vi "OAT Orbit Plot (Angle Waveform).vi"(0 "angle waveform (X and Y)":cluster{"r0":dbl, "dr":dbl, "Y":dbl[]}[](array[cluster]) {"r0" format="%.2p"; "dr" format="%.2p"; "Y" format="%.2f"}, 1 "orbit plot ref":refnum<vi>, 2 "reset? (T)":bool=TRUE, 3 "max axis display value":dbl format="%.2f", 5 "speed profile":T1 {"speed [RPM]" format="%.2f"; "time [s]" format="%.2f"}, 7 "interpolated pulse positions [s]":dbl[](array[numeric]) format="%.2f", 9 "revolutions to display":cluster{"start [rev]":dbl, "duration [rev]":dbl}={"start [rev]"=0.0, "duration [rev]"=1.0} {"duration [rev]" format="%.2f"; "start [rev]" format="%.2f"}, 11 "error in (no error)":errorcluster, 12 "rotating settings":T2={"shaft rotating direction"=0, "probe orientation"={"X (red)"=0, "Y (blue)"=90}} {"shaft rotating direction" items=["CCW", "CW"]}, 14 "trigger pulse direction":u16(ring)=1 items=["positive going", "negative going"]) -> (4 "orbit plot":T3, 15 "error out":errorcluster)   [LabVIEW 2017]
doc: "Draws an orbit plot of waveform signals on an XY graph. You can use sampled or resampled waveform signals from proximity transducers. You can use this polymorphic VI to draw an orbit plot of resampled signals or waveform signals. The data type you wire to the <B>resampled signals (X and Y)</B> determines the polymorphic instance to use."
uses:
  <vilib>/addons/Sound and Vibration/Order Analysis/Backward Compatibility/SubVIs/oa_Orbit Plot Control.ctl
  <vilib>/addons/Sound and Vibration/Order Analysis/Tach Process/SubVIs/speed profile.ctl
  <vilib>/addons/Sound and Vibration/Order Analysis/Resample Order Tracking/SoundVib_Resampling.lvlib
  <vilib>/addons/Sound and Vibration/Order Analysis/Tach Process/SoundVib_TachProcess.lvlib
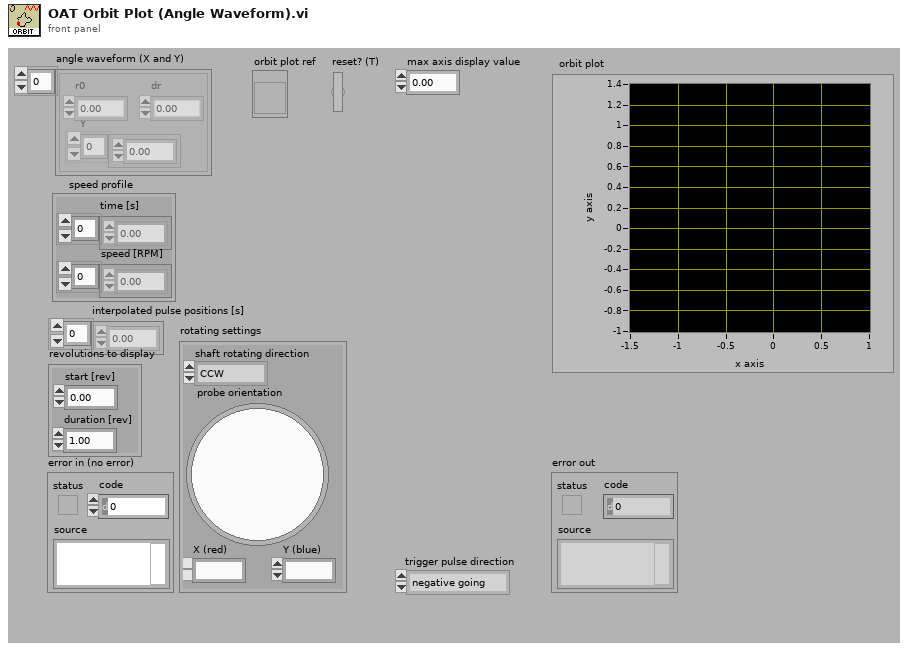
[diagram p1: front panel]
types:
  T1 = typedef "SoundVib_TachProcess.lvlib/speed profile.ctl" = cluster{"time [s]":dbl[], "speed [RPM]":dbl[]}
  T2 = cluster{"shaft rotating direction":u16, "probe orientation":cluster{"X (red)":u32, "Y (blue)":u32}}
  T3 = typedef "oa_Orbit Plot Control.ctl" = cluster{dbl[], dbl[]}[]
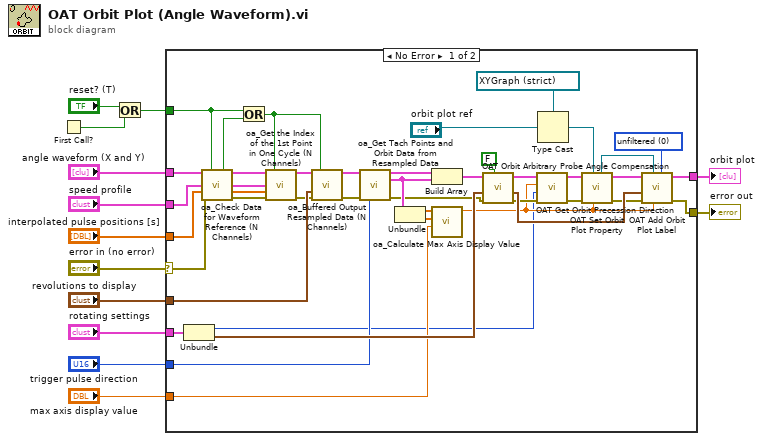
[diagram p0: block diagram]
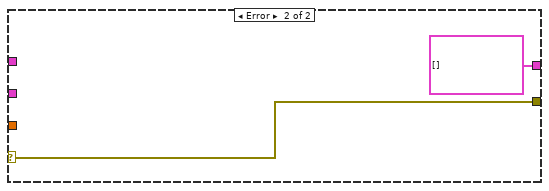
[diagram p2: hidden frame]
diagram:
  n1 = First Call?() -> (First Call?: T/F=w7:bool)
  n2 = Or(x="reset? (T)", y=w7) -> (x .or. y?=w6:bool)
  n3 = case shown="No Error" "error in (no error)" {
    selector: "error in (no error)" -> [w51 w58]
    tunnel: [w17 w58] -> w12
    tunnel: "angle waveform (X and Y)" -> [w52 _]
    tunnel: "speed profile" -> [w50 _]
    tunnel: "interpolated pulse positions [s]" -> [w49 _]
    tunnel: w6 -> [w48 _]
    tunnel: "revolutions to display" -> [w45 _]
    tunnel: [w34 cluster{dbl[], dbl[]}[] [] ("XY plot data out")] -> w4
    tunnel: "rotating settings" -> [w33 _]
    tunnel: "trigger pulse direction" -> [w29 _]
    tunnel: "max axis display value" -> [w27 _]
    frame No Error {
      w35 = u16 0 items=["unfiltered", "filtered"] ("plot type")
      n4 = Unbundle(w33) -> ("shaft rotating direction"=w20:u16, "probe orientation"=w32:cluster{"X (red)":u32, "Y (blue)":u32})
      n5 = call <vilib>:"oa_Check Data for Waveform Reference (N Channels).vi"("resampled signal"=w52, "reset? (True)"=w48, "speed profile"=w50, "interpolated pulse positions"=w49, "error in (no error)"=w51) -> ("reset"=w47:bool, "resampled data out"=w55:cluster{"r0":dbl, "dr":dbl, "Y":dbl[]}[], "speed profile out"=w53:T1, "interpolated pulse positions out"=w54:dbl[], "error out"=w56:errorcluster)  [unwired: 3 in, 3 out]
      n6 = Or(x=w48, y=w47) -> (x .or. y?=w43:bool)
      n7 = call <vilib>:"oa_Get the Index of the 1st Point in One Cycle (N Channels).vi"("resampled signal"=w55, "reset? (True)"=w43, "speed profile"=w53, "interpolated pulse positions"=w54, "error in (no error)"=w56) -> ("resampled signal out"=w46:cluster{"r0":dbl, "dr":dbl, "Y":dbl[]}[], "error out"=w44:errorcluster)  [unwired: 8 in, 1 out]
      n8 = call <vilib>:"oa_Buffered Output Resampled Data (N Channels).vi"("resampled signal in"=w46, "reset? (True)"=w43, "display revolutions"=w45, "error in"=w44) -> ("resampled signal out"=w31:cluster{"r0":dbl, "dr":dbl, "Y":dbl[]}[], "error out"=w30:errorcluster)  [unwired: 9 in, 1 out]
      n9 = call <vilib>:"oa_Get Tach Points and Orbit Data from Resampled Data.vi"("resampled signal in"=w31, "error in"=w30, "trigger pulse direction"=w29) -> ("tach points"=w28:cluster{dbl[], dbl[]}, "orbit"=w26:cluster{dbl[], dbl[]}, "error out"=w23:errorcluster)  [unwired: 10 in]
      n10 = Unbundle(w26) -> (w25:dbl[], w24:dbl[])
      n11 = Build Array(w28, w26) -> (w38:cluster{dbl[], dbl[]}[])
      n12 = call <vilib>:"oa_Calculate Max Axis Display Value.vi"("max axis display value in"=w27, "orbit data Y"=w24, "orbit data X"=w25) -> ("max data value out"=w21:dbl)  [unwired: 8 in]
      n13 = call <vilib>:"OAT Orbit Arbitrary Probe Angle Compensation.vi"("select methods"=FALSE, "error in (no error)"=w23, "probe angle"=w32, "XY plot data in"=w38) -> ("error out"=w22:errorcluster, "probe angle out"=w37:cluster{"X (red)":dbl, "Y (blue)":dbl}, "XY plot data out"=w42:cluster{dbl[], dbl[]}[])  [unwired: 5 in]
      n14 = call <vilib>:"OAT Get Orbit Precession Direction.vi"("error in (no error)"=w22, "shaft rotating direction"=w20, "max data value"=w21, "XY plot data in"=w42) -> ("error out"=w19:errorcluster, "XY plot data out"=w41:cluster{dbl[], dbl[]}[])  [unwired: 6 in]
      n15 = Type Cast(type=refnum<vi> refnum ("orbit plot ref"), x="orbit plot ref") -> (*(type *) &x=w14:refnum<vi>)
      n16 = call <vilib>:"OAT Set Orbit Plot Property.vi"("max value"=w21, "orbit plot ref"=w14, "error in (no error)"=w19, "XY plot data in"=w41) -> ("error out"=w18:errorcluster, "XY plot data out"=w40:cluster{dbl[], dbl[]}[], "orbit plot ref"=w39:refnum<vi>)  [unwired: 5 in]
      n17 = call <vilib>:"OAT Add Orbit Plot Label.vi"("plot type"=w35, "max value"=w21, "orbit plot ref"=w39, "error in (no error)"=w18, "probe angle out"=w37, "XY plot data in"=w40) -> ("error out"=w17:errorcluster, "XY plot data out"=w34:cluster{dbl[], dbl[]}[])  [unwired: 4 in]
    }
    frame Error {
    }
  }
  "orbit plot" <- w4
  "error out" <- w12
